vi "(format specifier)string function3.vi"() -> ()   [LabVIEW 2019]
panel:
  out "Resulting string":string
  in  "Numeric 2":u64=36
  in  "Numeric 1":u64=4567
  in  "String":string="O+ve"
  in  "Num 4":u32=53
  in  "Float":fxp<+/-,64,32>=167.54000000003725
  in  "Num 3":u32=1999
  in  "Num2":u32=11
  out "Resulting string":string
  in  "Num1":u32=13
  in  "String":string="Nagpur"
  in  "String":string="Falguni Suroshe"
  in  "String":string="name"
  # "String Function"
  # "5) Format Specifiers"
  # "Octadecimal format specifier"
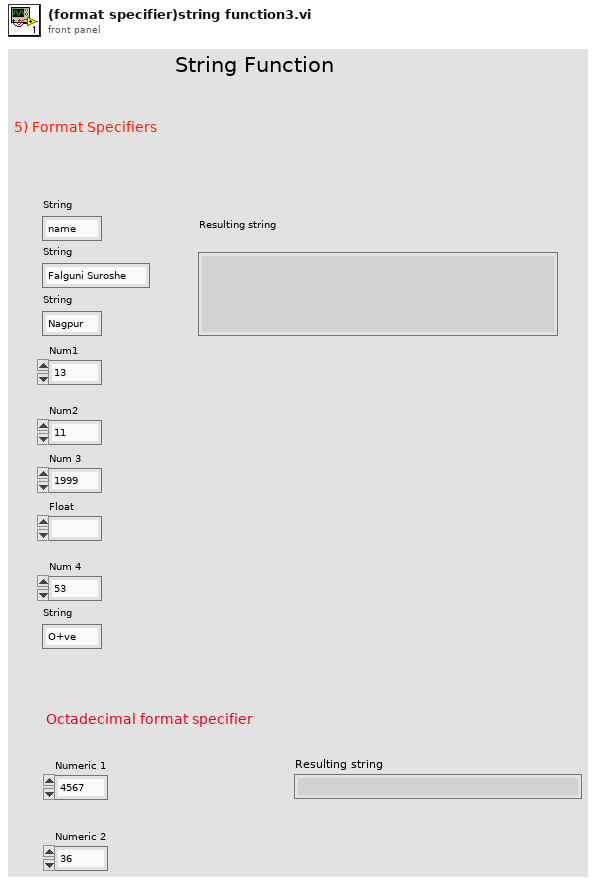
[diagram p1: front panel]
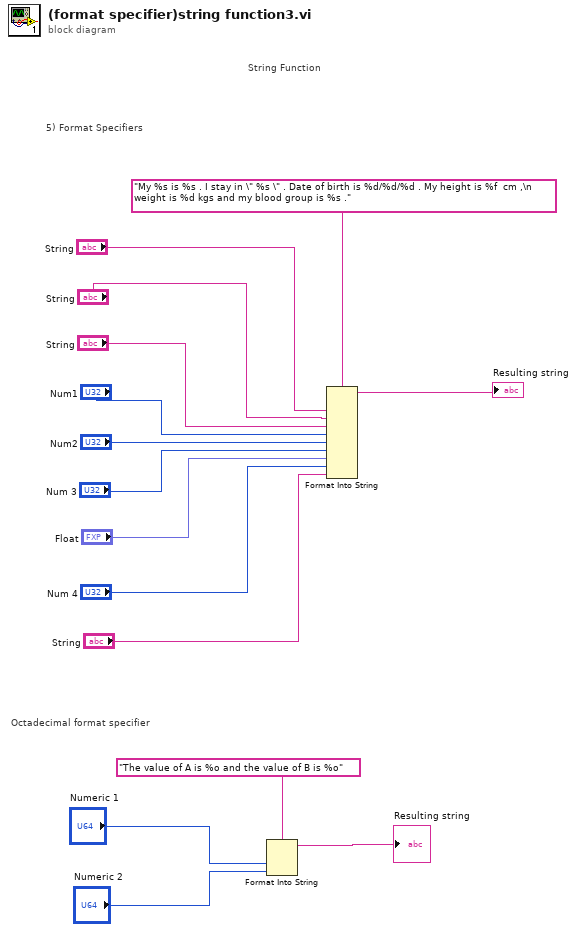
[diagram p0: block diagram]
diagram:
  # "Octadecimal format specifier"
  # "5) Format Specifiers"
  # "String Function"
  n1 = Format Into String(format string="The value of A is %o and the value of B is %o", "Numeric 1", "Numeric 2") -> (resulting string=→"Resulting string":string)  [unwired: 2 in, 1 out]
  n2 = Format Into String(format string="My %s is %s . I stay in \" %s \" . Date of birth is %d/%d/%d . My height is %f  cm ,\n weight is %d kgs and my blood group is %s .", "String", "String", "String", "Num1", "Num2", "Num 3", "Float", "Num 4", "String") -> (resulting string=→"Resulting string":string)  [unwired: 2 in, 1 out]
